vi "Set Dev Point.vi"(8 "error in (no error)":errorcluster, 9 "firmware revision":string(combo), 10 "dev point":T1={"dev point cap (100)"=100.0, "dev point loss (0)"=0.0}, 11 "VISA resource name":refnum<visa-resource-name>) -> (0 "error out":errorcluster, 2 "bridge error":T2, 3 "VISA resource name out":refnum<visa-resource-name>)   [LabVIEW 2019, in "Andeen-Hagerling 2700A.lvlib"]
doc: "Sets the capacitance and loss values for the Deviation Setpoint."
uses:
  Andeen-Hagerling 2700A.lvlib
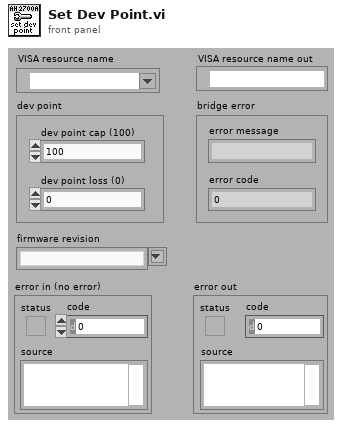
[diagram p1: front panel]
types:
  T1 = cluster{"dev point cap (100)":dbl, "dev point loss (0)":dbl}
  T2 = cluster{"error message":string, "error code":i32}
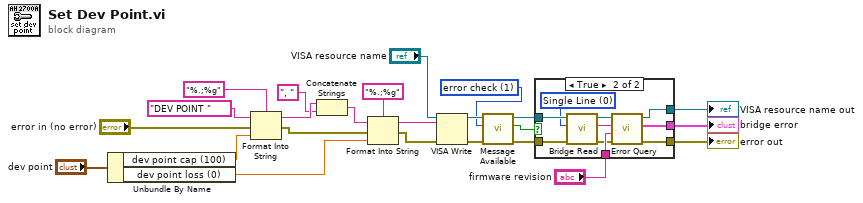
[diagram p0: block diagram]
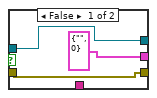
[diagram p2: hidden frame]
diagram:
  w1 = u16 1 items=["none", "error check", "multiline read", "infinite"] ("delay")
  n1 = Unbundle By Name("dev point") -> ("dev point cap (100)"=w3:dbl, "dev point loss (0)"=w2:dbl)
  n2 = Format Into String(format string="%.;%g", initial string="DEV POINT " ("command"), error in="error in (no error)", w3) -> (resulting string=w21:string, error out=w22:errorcluster)
  n3 = Concatenate Strings(w21, ", " ("command")) -> (w15:string)
  n4 = Format Into String(format string="%.;%g", initial string=w15, error in=w22, w2) -> (resulting string=w17:string, error out=w18:errorcluster)
  n5 = VISA Write(VISA resource name="VISA resource name", write buffer=w17, error in (no error)=w18) -> (VISA resource name out=w9:refnum<visa-resource-name>, error out=w8:errorcluster)  [unwired: 1 out]
  n6 = call "Message Available.vi"("error in (no error)"=w8, "delay"=w1, "VISA resource name"=w9) -> ("error out"=w11:errorcluster, "message available"=w13:bool, "VISA resource name out"=w12:refnum<visa-resource-name>)  [unwired: 6 in]
  n7 = case shown="True" w13 {
    tunnel: w12 -> [w26 w33]
    tunnel: w11 -> [w27 w32]
    tunnel: "firmware revision" -> [_ w37]
    tunnel: [w27 w36] -> w6
    tunnel: [w26 w35] -> w7
    tunnel: [T2 {"error message"="", "error code"=0} ("bridge error") w34] -> w5
    frame False {
    }
    frame True {
      w28 = u16 0 items=["Single Line", "Multi-Line"] ("Multiline")
      n8 = call "Bridge Read.vi"("error in (no error)"=w32, "multiline"=w28, "VISA resource name"=w33) -> ("error out"=w29:errorcluster, "read buffer"=w30:string, "VISA resource name out"=w31:refnum<visa-resource-name>)  [unwired: 6 in]
      n9 = call "Error Query.vi"("error in (no error)"=w29, "firmware revision"=w37, "measurement line"=w30, "VISA resource name"=w31) -> ("error out"=w36:errorcluster, "bridge error"=w34:T2, "VISA resource name out"=w35:refnum<visa-resource-name>)  [unwired: 5 in]
    }
  }
  "VISA resource name out" <- w7
  "error out" <- w6
  "bridge error" <- w5
